vi "2a_Datalog write.vi"() -> ()   [LabVIEW 2010]
panel:
  out "Numeric":i32
  in  "Header":string
  out "?":dbl[][](graph)
  in  "Cluster":T1
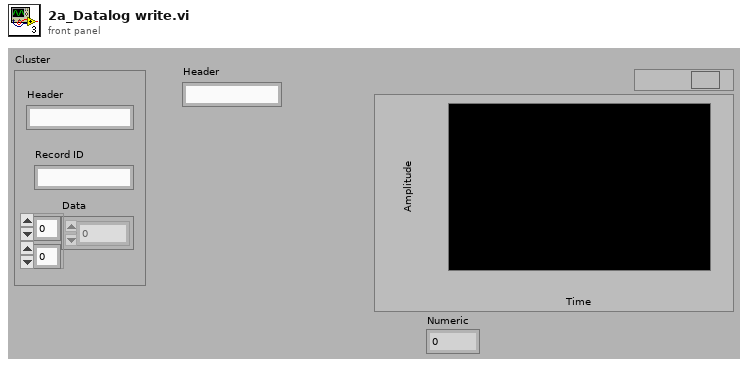
[diagram p1: front panel]
types:
  T1 = cluster{"Data":dbl[][], "Header":string, "Record ID":string}
  T2 = enum16{"open", "replace", "create", "open or create", "replace or create", "replace or create with confirmation"}
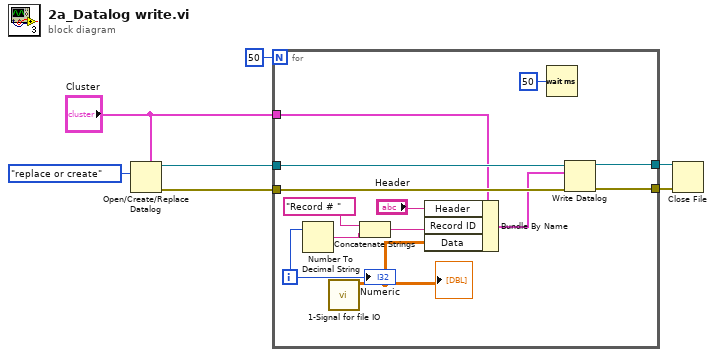
[diagram p0: block diagram]
diagram:
  n1 = Open/Create/Replace Datalog(5:"Cluster", 10:T2."replace or create" ("operation (0:open)")) -> (0:w2:errorcluster, 3:w3:refnum<k1>)  [unwired: 4 in, 1 out]
  n2 = for {
    N: 50 -> [_]
    tunnel: w3 -> [w19]
    tunnel: w2 -> [w18]
    tunnel: [w17] -> w6
    tunnel: [w16] -> w5
    tunnel: "Cluster" -> [w15]
    i -> [w14]
    n3 = Number To Decimal String(number=w14) -> (decimal integer string=w13:string)  [unwired: 1 in]
    n4 = call "1-Signal for file IO.vi"() -> ("Data"=w8:dbl[][])  [unwired: 10 in]
    "?" <- w8
    n5 = Concatenate Strings("Record # " ("string"), w13) -> (w11:string)
    n6 = Bundle By Name(cluster=w15, "Header"="Header", "Record ID"=w11, "Data"=w8) -> (w9:T1)
    n7 = Wait (ms)(milliseconds to wait=u32 50) -> ()  [unwired: 1 out]
    n8 = Write Datalog(4:w18, 6:w9, 7:w19) -> (0:w17:errorcluster, 3:w16:refnum<k1>)
    "Numeric" <- w14
  }
  n9 = Close File(refnum=w5, error in=w6) -> ()  [unwired: 2 out]
